vi "Interpret_Read Coils.vi"(8 "error in (no error)":errorcluster, 10 "MB_PDU_req in":T1={"Function Code"=1, "Data"=[], "RTU_DataBytes"=0}, 11 "MB_PDU_resp in":T1={"Function Code"=1, "Data"=[], "RTU_DataBytes"=0}) -> (0 "error out":errorcluster, 2 "Coils":bool[](array[boolean]))   [LabVIEW 2016, in "MB Master.lvlib"]
doc: "Extracts the data of a PDU request/response pair based on the function code of the response.\n\nReturns an array of booleans for coils and discrete inputs.\nReturns an array of unsigned 16-bit integers for input and holding registers."
uses:
  MB Master.lvlib
  MB_PDU_Cluster.ctl
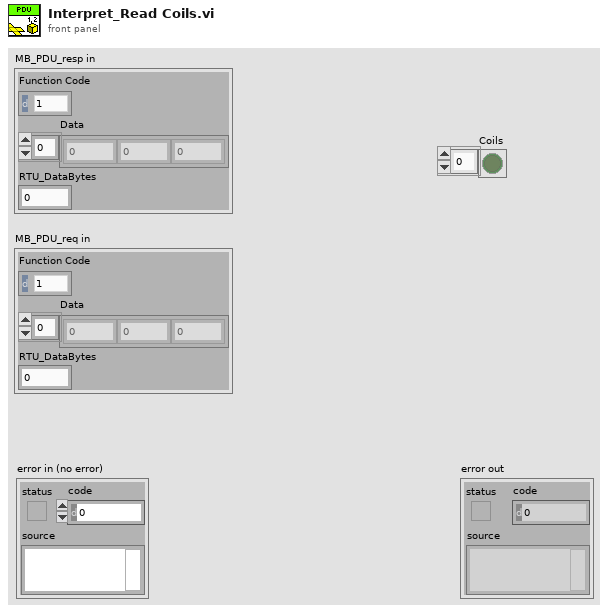
[diagram p1: front panel]
types:
  T1 = typedef "MB Master.lvlib/MB_PDU_Cluster.ctl" = cluster{"Function Code":u8, "Data":u8[], "RTU_DataBytes":i32}
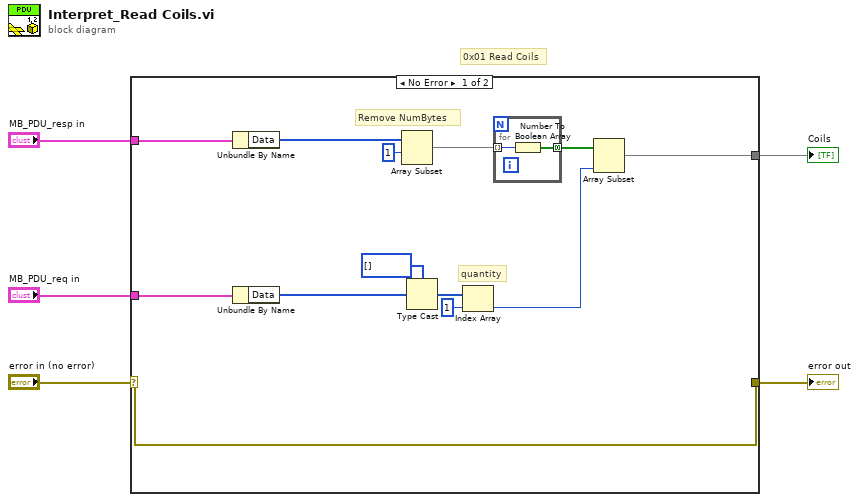
[diagram p0: block diagram]
diagram:
  # "0x01 Read Coils"
  n1 = case shown="No Error" "error in (no error)" {
    selector: "error in (no error)" -> [w18 w21]
    tunnel: [w18 w21] -> w4
    tunnel: "MB_PDU_resp in" -> [w17 _]
    tunnel: "MB_PDU_req in" -> [w15 _]
    tunnel: [w13 _] -> w1
    frame No Error {
      # "Remove NumBytes"
      # "quantity"
      n2 = Unbundle By Name(w17) -> ("Data"=w16:u8[])
      n3 = Unbundle By Name(w15) -> ("Data"=w14:u8[])
      n4 = Array Subset(array=w16, index=1) -> (w11:u8[])  [unwired: 1 in]
      n5 = Type Cast(type=u16[] [], x=w14) -> (*(type *) &x=w8:u16[])
      n6 = Index Array(array=w8, index=1) -> (element=w6:u16)
      n7 = for {
        tunnel: w11 -> [w20] mode=indexing
        tunnel: [w19] -> w10 mode=concatenating
        n8 = Number To Boolean Array(number=w20) -> (Boolean array=w19:bool[])
      }
      n9 = Array Subset(array=w10, length=w6) -> (w13:bool[])  [unwired: 1 in]
    }
    frame Error {
    }
  }
  "error out" <- w4
  "Coils" <- w1
